vi "Close.vi"(11 "FpgaRef5761 In":refnum<class "FpgaRef5761.lvclass">) -> ()   [LabVIEW 2018, in "FpgaRef5761.lvclass"]
uses:
  FpgaRef5761.lvclass
  FpgaRef5761.lvclass/FpgaRef5761.ctl
  <vilib>/FPGAPlugInAG/Dynamic/niLvFpga_Close_Dynamic.vi
  FpgaRefBase/FpgaRefBase.lvclass
  <vilib>/rvi/interface/nirviCloseFPGA/nirviCloseFPGA.xnode
  5761 FPGA ref.ctl
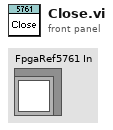
[diagram p1: front panel]
types:
  T1 = typedef "5761 FPGA ref.ctl" = refnum<k20>
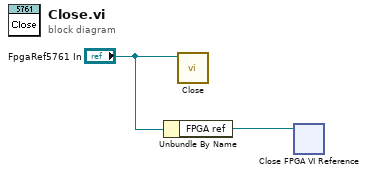
[diagram p0: block diagram]
diagram:
  n1 = Unbundle By Name("FpgaRef5761 In") -> ("FPGA ref"=w1:T1)
  n2 = call-parent "Close.vi"("FpgaRefBase In"="FpgaRef5761 In") -> ()  [unwired: 11 in]
  n3 = xnode "Close FPGA VI Reference"("FPGA VI Reference In"=w1) -> ()  [unwired: 1 in, 1 out]
